vi "Tolerance.vi"(1 "Tolerance":dbl, 2 "Input":dbl) -> (0 "Output":dbl)   [LabVIEW 2014]
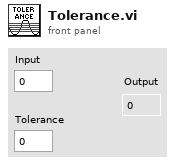
[diagram p1: front panel]
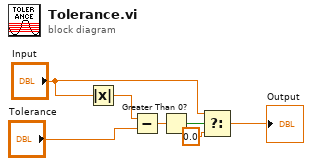
[diagram p0: block diagram]
diagram:
  n1 = Absolute Value(x="Input") -> (abs(x)=w7:dbl)
  n2 = Subtract(x=w7, y="Tolerance") -> (x-y=w6:dbl)
  n3 = Greater Than 0?(x=w6) -> (x > 0?=w5:bool)
  n4 = Select(t="Input", s=w5, f=0.0) -> (s? t:f=→"Output":dbl)
